vi "CaLabGet.vi"   [LabVIEW 2018]
doc: "This is a VI for getting values of EPICS variables.\n\n<b>INPUT:</b>\n <b>PV Name(s)</b>\n Name of EPICS variable OR string array of EPICS variable names \n Attention: Mixed target data types arise as a result of a 2-D array of size\n (number of names) * (size of largest data type)!\n <b>Field Names</b>\n Optional\n String array of static EPICS fields (\"EGU\", \"DESCRIPTION\" etc.)\n <b>Timeout (3)</b>\n Optional\n Timeout for Channel Access requests in seconds\n Default value: 3 seconds\n <b>NoMDEL (F)</b>\n * for use without pre-initialisation only\n optional\n true: ignore monitor dead-band of Channel Access (EPICS)\n <b>variable PV names (F)</b>\n * for use without pre-initialisation only\n optional\n true: in case of changing PV names at PV name input (performance drop)\n <b>Error in (no error)</b>\n\n<b>OUTPUT:</b>\n <b>PV Name(s) (dup)</b>\n Name of EPICS variable OR string array of EPICS variable names\n <b>1st Value(s)</b>\n Value of variable as String OR string array\n Shows first item of value array only\n <b>1st Value(s)</b>\n Value of variable as Double or double array\n Shows first item of value array only\n <b>Value array(s)\n All values of variable in Double array (1D / 2D)</b>\n <b>PV Info / PV Info array</b>\n <b>Status</b>\n FALSE: request(s) successful\n TRUE: warnings or errors\n <b>Error out</b>\n Global io error"
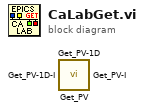
[diagram p0: block diagram]
diagram:
  n1 = call <userlib>:"Get_PV.vi"() -> ()  [unwired: 9 in, 7 out]
  n2 = call <userlib>:"Get_PV-1D.vi"() -> ()  [unwired: 9 in, 7 out]
  n3 = call <userlib>:"Get_PV-1D-I.vi"() -> ()  [unwired: 9 in, 7 out]
  n4 = call <userlib>:"Get_PV-I.vi"() -> ()  [unwired: 9 in, 7 out]
